vi "DELETE getWFMQueueRefnum.vi"(8 "error in (no error)":errorcluster, 10 "wait for min buffer?":bool, 11 "DAQmx in":refnum<class "DAQmx.lvclass">) -> (0 "error out":errorcluster, 1 "timed out?":bool, 2 "AO":waveform(dbl)[](array[waveform]), 3 "DAQmx out":refnum<class "DAQmx.lvclass">, 4 "REF_Y":waveform(dbl)[](array[waveform]), 6 "REF_X":waveform(dbl)[](array[waveform]))   [LabVIEW 2019]
uses:
  DAQmx/DAQmx.lvclass
  <vilib>/ErrorRing/Error Ring.xnode
  <vilib>/Utility/error.llb/Error Cluster From Error Code.vi
  C:/Program Files/National Instruments/LabVIEW 2019/vi.lib/JKI/JKI SMO/SMO/SMO.lvclass
panel:
  out "v timed out":bool
  out "AO queue #":i32
  out "Y /empty":bool
  out "X /empty":bool
  out "AO /empty":bool
  out "^ /empty":bool
  out "time waiting for buffer":dbl format="%#_6p"
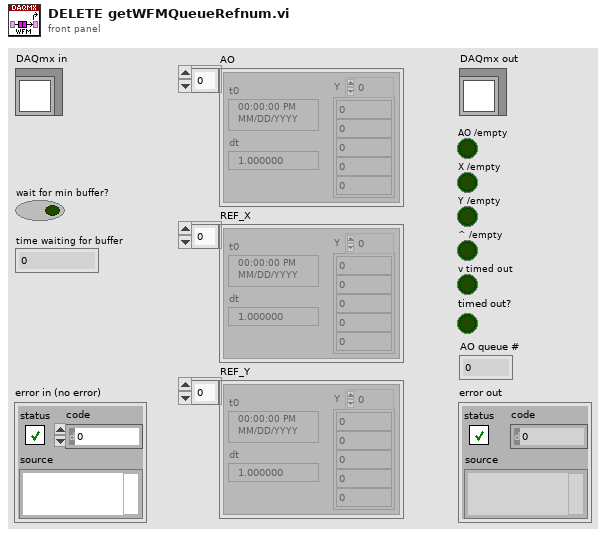
[diagram p1: front panel]
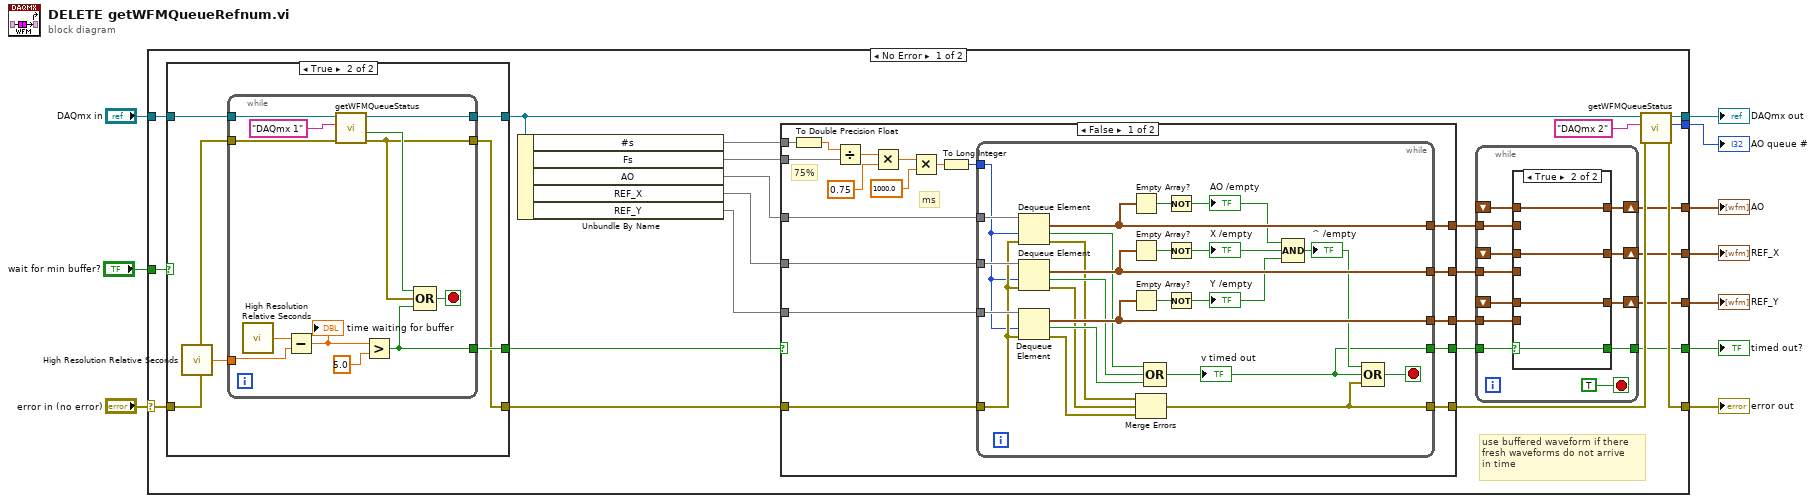
[diagram p0: block diagram]
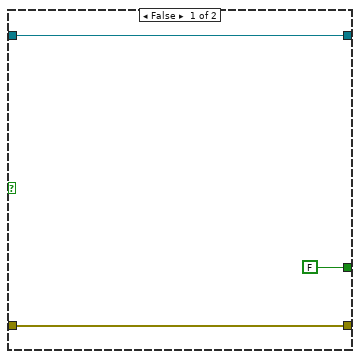
[diagram p2: hidden frame]
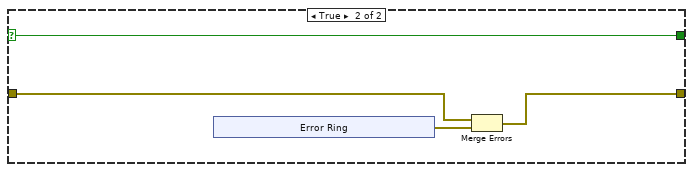
[diagram p3: hidden frame]
diagram:
  n1 = case shown="No Error" "error in (no error)" {
    selector: "error in (no error)" -> [w29 w127]
    tunnel: [w22 w127] -> w2
    tunnel: [w24 w126] -> w10
    tunnel: "DAQmx in" -> [w31 w126]
    tunnel: [w13 _] -> w9
    tunnel: [w12 _] -> w4
    tunnel: [w15 _] -> w8
    tunnel: [w17 _] -> w7
    tunnel: "wait for min buffer?" -> [w27 _]
    tunnel: [w20 _] -> w1
    frame No Error {
      # "use buffered waveform if there\nfresh waveforms do not arrive\nin time"
      n2 = case shown="True" w27 {
        tunnel: [w35 w43] -> w25
        tunnel: w31 -> [w35 w42]
        tunnel: [FALSE w41] -> w30
        tunnel: w29 -> [w36 w40]
        tunnel: [w36 w39] -> w28
        frame False {
        }
        frame True {
          n3 = call <vilib>:"High Resolution Relative Seconds.vi"() -> ("relative seconds"=w38:dbl)
          n4 = while {
            tunnel: w38 -> [w45]
            tunnel: [w50] -> w41
            tunnel: w40 -> [w49]
            tunnel: [w48] -> w39
            tunnel: w42 -> [w54]
            tunnel: [w55] -> w43
            stop <- w51 stop-if-true
            n5 = call <vilib>:"High Resolution Relative Seconds.vi"() -> ("relative seconds"=w46:dbl)
            n6 = Subtract(x=w46, y=w45) -> (x-y=w44:dbl)
            "time waiting for buffer" <- w44
            n7 = call "getWFMQueueStatus.vi"("error in (no error)"=w49, "instance"="DAQmx 1", "DAQmx in"=w54) -> ("error out"=w48:errorcluster, "Min Queue Filled"=w52:bool, "DAQmx out"=w55:refnum<class "DAQmx.lvclass">)  [unwired: 5 in, 1 out]
            n8 = Greater?(x=w44, y=5.0) -> (0:w50:bool)
            n9 = Compound Arithmetic op=OR(w52, w48, w50) -> (w51:bool)
          }
        }
      }
      n10 = Unbundle By Name(w25) -> ("#s"=w11, "Fs"=w21, "AO"=w34, "REF_X"=w32, "REF_Y"=w33)
      n11 = case shown="False" w30 {
        selector: w30 -> [_ w98]
        tunnel: [w73 w98] -> w18
        tunnel: [w72 w100] -> w23
        tunnel: [w71 _] -> w19
        tunnel: [w70 _] -> w16
        tunnel: [w69 _] -> w14
        tunnel: w34 -> [w68 _]
        tunnel: w32 -> [w67 _]
        tunnel: w33 -> [w66 _]
        tunnel: w28 -> [w65 w99]
        tunnel: w21 -> [w63 _]
        tunnel: w11 -> [w60 _]
        frame False {
          # "ms"
          # "75%"
          n12 = To Double Precision Float(number=w60) -> (double precision float=w59:dbl)
          n13 = Divide(x=w59, y=w63) -> (x/y=w64:dbl)
          n14 = Multiply(x=w64, y=0.75 ("timeout in ms (-1)")) -> (x*y=w58:dbl)
          n15 = Multiply(x=w58, y=1000.0 ("timeout in ms (-1)")) -> (x*y=w57:dbl)
          n16 = To Long Integer(number=w57) -> (32bit integer=w61:i32)
          n17 = while {
            tunnel: [w74] -> w73
            tunnel: [w79] -> w72
            tunnel: w68 -> [w97]
            tunnel: w67 -> [w96]
            tunnel: w66 -> [w95]
            tunnel: [w84] -> w71
            tunnel: [w85] -> w70
            tunnel: [w94] -> w69
            tunnel: w65 -> [w86]
            tunnel: w61 -> [w83]
            stop <- w90 stop-if-true
            n18 = Dequeue Element(queue=w97, timeout in ms (-1)=w83, error in (no error)=w86) -> (element=w84:waveform(dbl)[], timed out?=w82:bool, error out=w80:errorcluster)  [unwired: 1 out]
            n19 = Dequeue Element(queue=w96, timeout in ms (-1)=w83, error in (no error)=w86) -> (element=w85:waveform(dbl)[], timed out?=w89:bool, error out=w87:errorcluster)  [unwired: 1 out]
            n20 = Dequeue Element(queue=w95, timeout in ms (-1)=w83, error in (no error)=w86) -> (element=w94:waveform(dbl)[], timed out?=w88:bool, error out=w81:errorcluster)  [unwired: 1 out]
            n21 = Empty Array?(array=w84) -> (empty?=w93:bool)
            n22 = Empty Array?(array=w85) -> (empty?=w92:bool)
            n23 = Empty Array?(array=w94) -> (empty?=w91:bool)
            n24 = Merge Errors(w80, w87, w81) -> (w79:errorcluster)
            n25 = Compound Arithmetic op=OR(w82, w89, w88) -> (w74:bool)
            "v timed out" <- w74
            n26 = Not(x=w93) -> (.not. x?=w75:bool)
            "AO /empty" <- w75
            n27 = Not(x=w92) -> (.not. x?=w77:bool)
            "X /empty" <- w77
            n28 = Not(x=w91) -> (.not. x?=w76:bool)
            "Y /empty" <- w76
            n29 = Compound Arithmetic op=AND(w75, w77, w76) -> (w78:bool)
            "^ /empty" <- w78
            n30 = Compound Arithmetic op=OR(w78, w74, w79) -> (w90:bool)
          }
        }
        frame True {
          n31 = xnode "Error Ring"() -> ("error out"=w101:errorcluster)
          n32 = Merge Errors(w99, w101) -> (w100:errorcluster)
        }
      }
      n33 = while {
        tunnel: w19 -> [w114]
        shift-right: [w115] -> w13
        shift-left: _ -> [w107]
        tunnel: w18 -> [w116]
        tunnel: w16 -> [w112]
        shift-right: [w113] -> w17
        shift-left: _ -> [w108]
        tunnel: w14 -> [w110]
        shift-right: [w111] -> w15
        shift-left: _ -> [w109]
        tunnel: [w106] -> w12
        stop <- TRUE stop-if-true
        n34 = case shown="True" w116 {
          selector: w116 -> [w118 w122]
          tunnel: [w121 w123] -> w115
          tunnel: w114 -> [w121 _]
          tunnel: [w120 w124] -> w113
          tunnel: w112 -> [w120 _]
          tunnel: [w119 w125] -> w111
          tunnel: w110 -> [w119 _]
          tunnel: w109 -> [_ w125]
          tunnel: w108 -> [_ w124]
          tunnel: w107 -> [_ w123]
          tunnel: [w118 w122] -> w106
          frame False {
          }
          frame True {
          }
        }
      }
      n35 = call "getWFMQueueStatus.vi"("error in (no error)"=w23, "instance"="DAQmx 2", "DAQmx in"=w25) -> ("error out"=w22:errorcluster, "AO queue #"=w20:i32, "DAQmx out"=w24:refnum<class "DAQmx.lvclass">)  [unwired: 5 in, 1 out]
    }
    frame Error {
    }
  }
  "error out" <- w2
  "DAQmx out" <- w10
  "AO" <- w9
  "timed out?" <- w4
  "REF_X" <- w7
  "REF_Y" <- w8
  "AO queue #" <- w1
